vi "write to database.vi"(1 "2D data":string[][](array[string]) caption="二维数据", 2 "Header":string[](array[string]), 3 "error in (no error)":errorcluster caption="错误输入（无错误）", 4 "data in":string[](array[string]), 5 "file name":string, 6 "path":path) -> (0 "new file path (Not A Path if cancelled)":path caption="新建文件路径（取消时为非法路径）")   [LabVIEW 2018]
uses:
  <vilib>/Utility/file.llb/Write To Spreadsheet File (string).vi
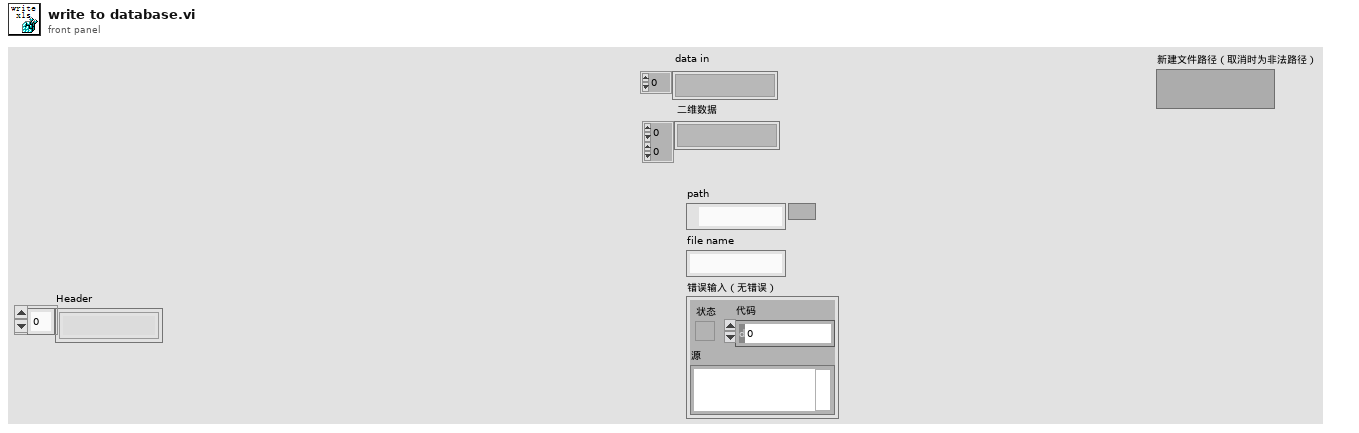
[diagram p1: front panel]
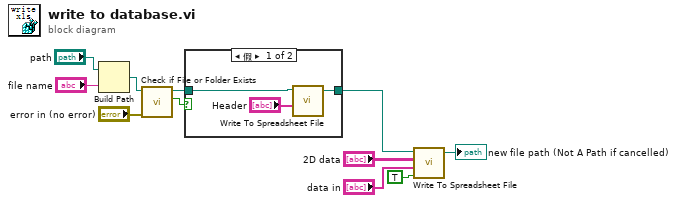
[diagram p0: block diagram]
diagram:
  n1 = Build Path(base path="path", name or relative path="file name") -> (appended path=w9:path)
  n2 = call <vilib>:"Check if File or Folder Exists.vi"("error in (no error)"="error in (no error)", "path"=w9) -> ("file or folder exists?"=w7:bool, "dup path"=w6:path)  [unwired: 7 in, 1 out]
  n3 = case shown="假" w7 {
    tunnel: [w13 w15] -> w5
    tunnel: w6 -> [w14 w15]
    frame False {
      n4 = call-poly <vilib>:"Write To Spreadsheet File.vi"("1D data"="Header", "file path (dialog if empty)"=w14) -> ("new file path (Not A Path if cancelled)"=w13:path)  [unwired: 6 in]
    }
    frame True {
    }
  }
  n5 = call-poly <vilib>:"Write To Spreadsheet File.vi"("append to file? (new file:F)"=TRUE, "1D data"="data in", "2D data"="2D data", "file path (dialog if empty)"=w5) -> ("new file path (Not A Path if cancelled)"=→"new file path (Not A Path if cancelled)":path)  [unwired: 4 in]
